vi "Module Cleanup.vi"(8 "error in (no error)":errorcluster, 11 "DAQmxDI in":refnum<class "DAQmxDI.lvclass">) -> (0 "error out":errorcluster, 3 "DAQmxDI out":refnum<class "DAQmxDI.lvclass">)   [LabVIEW 2020, in "VolatusDAQ.lvlib" / "DAQmxDI.lvclass"]
uses:
  DAQmxDI.lvclass
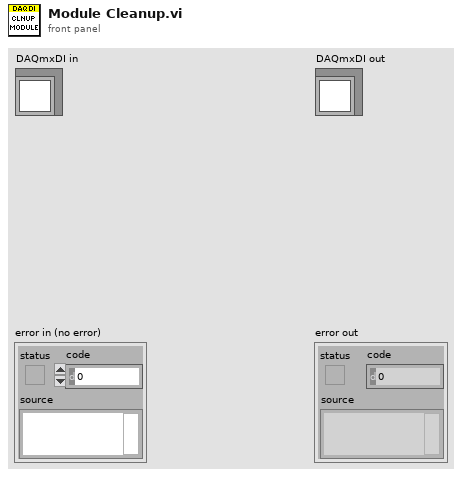
[diagram p1: front panel]
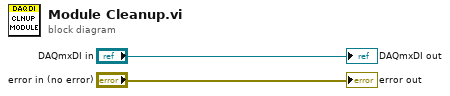
[diagram p0: block diagram]
diagram:
  "error out" <- "error in (no error)"
  "DAQmxDI out" <- "DAQmxDI in"
